vi "io_bin_data_instrument_to_PC.vi"(8 "error in":errorcluster, 10 "Query (none)":string, 11 "VISA resource name":refnum<visa-resource-name>) -> (0 "error out":errorcluster, 1 "Data Size":i32, 2 "String out":string, 3 "VISA resource name out":refnum<visa-resource-name>)   [LabVIEW 2014, in "rszvl_rsidr_core.lvlib"]
uses:
  rszvl_rsidr_core.lvlib
  type_Error_Codes.ctl
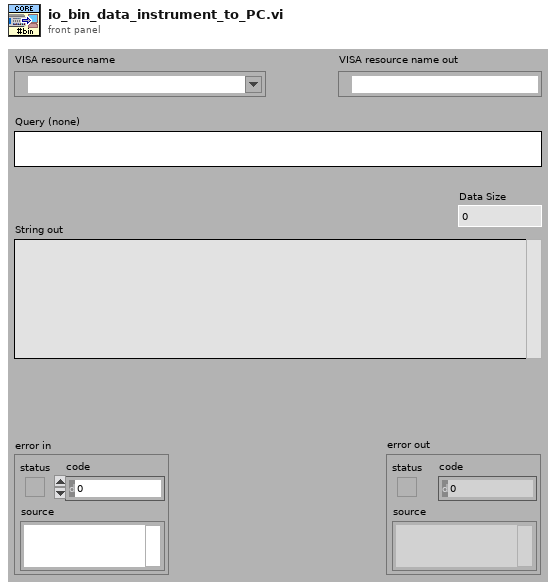
[diagram p1: front panel]
types:
  T1 = typedef "rszvl_rsidr_core.lvlib/type_Error_Codes.ctl" = enum16{"No_error", "VISA_err_ResourceNotFound", "VISA_err_Timeout", "VISA_warn_MoreDataAvailable", "RS_err_MissingCallback", "RS_err_InvalidAttribute", "RS_err_InvalidValue", "RS_err_UnknownResource", "RS_err_AlreadyInitialized", "RS_err_InstrumentStatus", "RS_err_BadRepCapName", "RS_err_TypesMismatch", "RS_err_ValueNotSupported", "RS_err_InvalidRngTable", "RS_err_IDqueryFail", "RS_err_UnexpResponse", "VISA_warn_ConfigNotLoaded", "RS_err_AttributeNotReadable", "RS_err_AttributeNotWritable", "RS_err_InstrumentType", "RS_err_InstrumentOption", "VISA_err_InvalidSize", "RS_err_ReliabilityIndicator", "VISA_warn_UnknownStatus", "VISA_warn_TermCharRead", "VISA_err_IO_error"}
  T2 = typedef "rszvl_rsidr_core.lvlib/type_Session_Data.ctl" = cluster{"Instr type":string, "Instr type for err. msg.":string, "Installed Options":string[], "OPC Timeout":i32, "Query Instrument Status":bool, "Check Range":bool, "Check Options":bool, "Add LF to Write":bool, "Simulate":bool, "Logging":bool, "Logging params":variant, "Interface Type":enum16{"Unknown", "GPIB", "VXI", "GPIB_VXI", "ASRL", "PXI", "TCPIP", "USB", "SOCKET"}, "Fast Sweep":i32, "AdditionalFlags":i32, "WaitBeforeWrite":i32, "WaitBeforeRead":i32, "BinDataChunkSize":i64}
  T3 = enum16{"Unknown", "GPIB", "VXI", "GPIB_VXI", "ASRL", "PXI", "TCPIP", "USB", "SOCKET"}
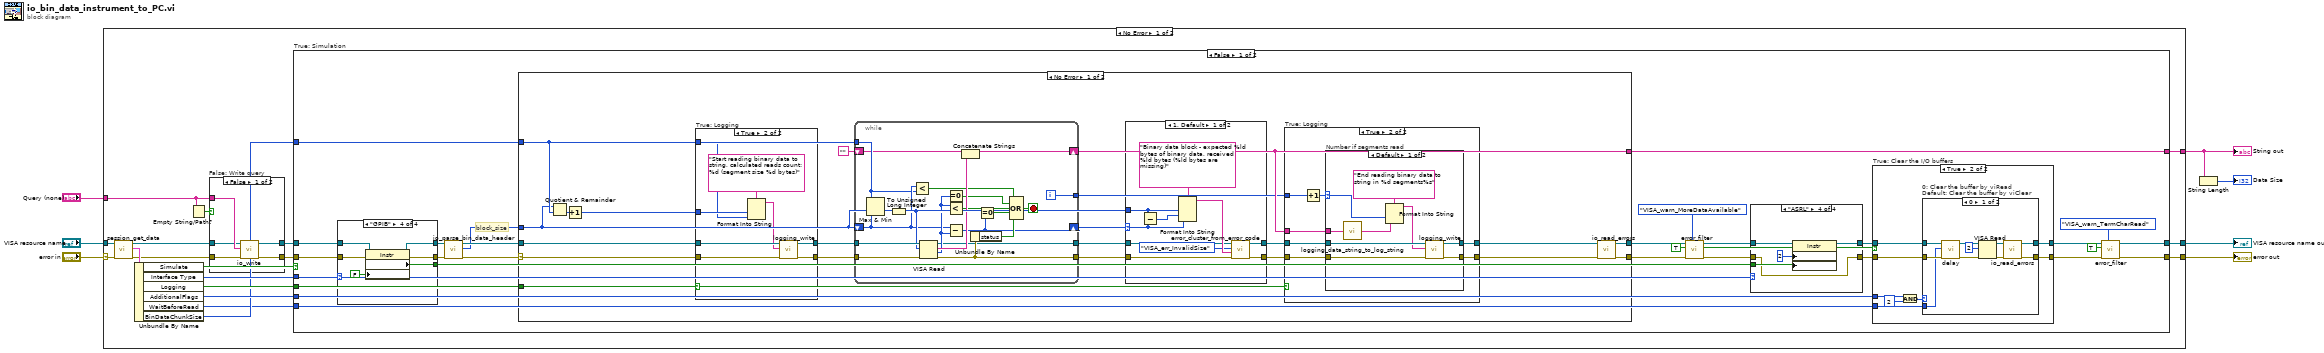
[diagram p0: block diagram]
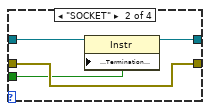
[diagram p4: hidden frame]
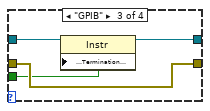
[diagram p5: hidden frame]
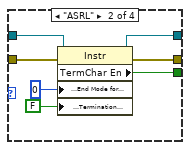
[diagram p7: hidden frame]
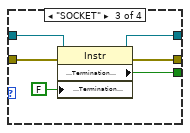
[diagram p8: hidden frame]
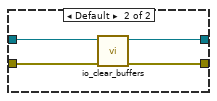
[diagram p10: hidden frame]
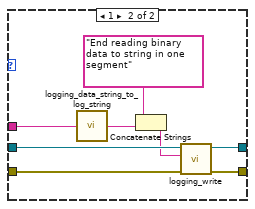
[diagram p12: hidden frame]
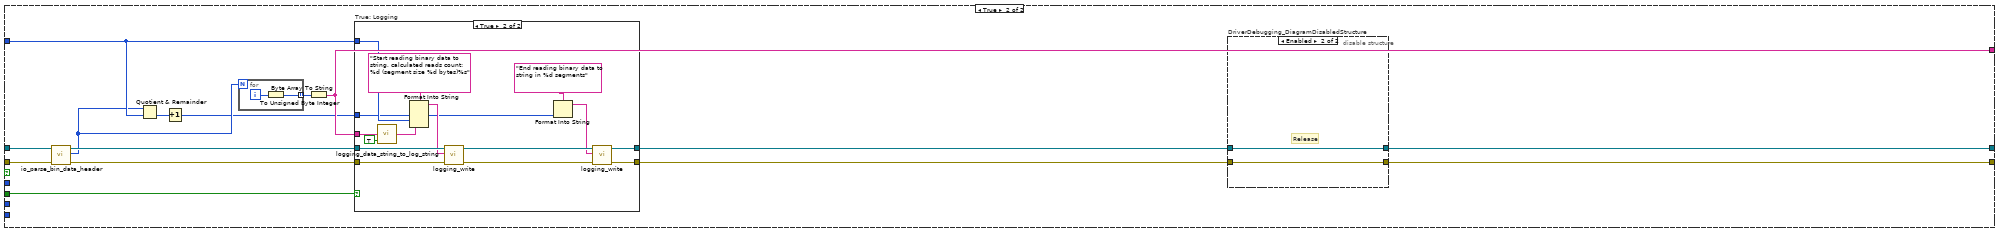
[diagram p16: hidden frame]
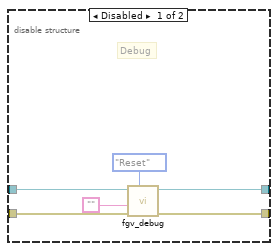
[diagram p18: hidden frame]
diagram:
  n1 = case shown="No Error" "error in" {
    selector: "error in" -> [w23 w256]
    tunnel: [w25 w255] -> w7
    tunnel: [w24 w256] -> w6
    tunnel: "VISA resource name" -> [w22 w255]
    tunnel: [w18 _] -> w2
    tunnel: "Query (none)" -> [w11 _]
    frame No Error {
      n2 = call "session_get_data.vi"("error in"=w23, "VISA resource name"=w22) -> ("error out"=w15:errorcluster, "Session User Data out"=w20:T2, "VISA resource name out"=w14:refnum<visa-resource-name>)  [unwired: 7 in]
      n3 = Unbundle By Name(w20) -> ("Simulate"=w21:bool, "Interface Type"=w19:T3, "Logging"=w17:bool, "AdditionalFlags"=w10:i32, "WaitBeforeRead"=w8:i32, "BinDataChunkSize"=w9:i64)
      n4 = Empty String/Path?(string/path=w11) -> (empty?=w16:bool)
      n5 = case "False: Write query" shown="False" w16 {
        tunnel: w15 -> [w29 w31]
        tunnel: [w27 w31] -> w13
        tunnel: [w26 w32] -> w12
        tunnel: w11 -> [w30 _]
        tunnel: w14 -> [w28 w32]
        frame False {
          n6 = call "io_write.vi"("error in"=w29, "write buffer"=w30, "VISA resource name"=w28) -> ("error out"=w27:errorcluster, "VISA resource name out"=w26:refnum<visa-resource-name>)  [unwired: 7 in]
        }
        frame True {
        }
      }
      n7 = case "True: Simulation" shown="False" w21 {
        tunnel: w13 -> [w48 w225]
        tunnel: w12 -> [w49 w226]
        tunnel: [w38 w214] -> w25
        tunnel: [w37 w215] -> w24
        tunnel: w19 -> [w53 _]
        tunnel: [w52 w219] -> w18
        tunnel: w17 -> [w51 w227]
        tunnel: w9 -> [w50 w222]
        tunnel: w10 -> [w47 _]
        tunnel: w8 -> [w33 _]
        frame False {
          # "block_size"
          n8 = case "4: ASRL" shown="\"GPIB\"" w53 {
            tunnel: w48 -> [w77 w84 w91 w97]
            tunnel: w49 -> [w78 w83 w90 w96]
            tunnel: [w78 w82 w89 w95] -> w57
            tunnel: [w77 w81 w88 w94] -> w58
            tunnel: [_ w79 w86 w92] -> w36
            frame Default {
            }
            frame "ASRL" {
              n9 = property on="Property Node" class="Instr"(reference=w83, error in=w84, "Serial Settings:End Mode for Reads"=u16 0 ("ASRL End In"), "Message Based Settings:Termination Character Enable"=FALSE ("TermChar En")) -> (reference out=w82:refnum<visa-resource-name>, error out=w81:errorcluster, "TermChar En"=w79:bool)
            }
            frame "SOCKET" {
              n10 = property on="Property Node" class="Instr"(reference=w90, error in=w91, "Message Based Settings:Termination Character Enable"=FALSE ("TermChar En")) -> (reference out=w89:refnum<visa-resource-name>, error out=w88:errorcluster, "Message Based Settings:Termination Character Enable"=w86:bool)
            }
            frame "GPIB" {
              n11 = property on="Property Node" class="Instr"(reference=w96, error in=w97, "Message Based Settings:Termination Character Enable"=FALSE ("TermChar En")) -> (reference out=w95:refnum<visa-resource-name>, error out=w94:errorcluster, "Message Based Settings:Termination Character Enable"=w92:bool)
            }
          }
          n12 = call "io_parse_bin_data_header.vi"("error in"=w58, "VISA resource name"=w57) -> ("error out"=w56:errorcluster, "Size of the bin data"=w54:i64, "VISA resource name out"=w55:refnum<visa-resource-name>)  [unwired: 6 in, 1 out]
          n13 = case shown="No Error" w56 {
            selector: w56 -> [w142 w212]
            tunnel: [w137 w212] -> w35
            tunnel: w55 -> [w141 w211]
            tunnel: w54 -> [w131 _]
            tunnel: w50 -> [w134 _]
            tunnel: [w136 w211] -> w34
            tunnel: [w135 _] -> w52
            tunnel: w51 -> [w140 _]
            frame No Error {
              n14 = Quotient & Remainder(x=w131, y=w134) -> (floor(x/y)=w139:i64)  [unwired: 1 out]
              n15 = Increment(x=w139) -> (x+1=w138:i64)
              n16 = case "True: Logging" shown="True" w140 {
                tunnel: w142 -> [w202 w208]
                tunnel: [w202 w210] -> w125
                tunnel: w141 -> [w201 w207]
                tunnel: [w201 w209] -> w126
                tunnel: w134 -> [_ w203]
                tunnel: w138 -> [_ w204]
                frame False {
                }
                frame True {
                  n17 = Format Into String(format string="Start reading binary data to string, calculated reads count: %d (segment size %d bytes)", w204, w203) -> (resulting string=w205:string)  [unwired: 2 in, 1 out]
                  n18 = call "logging_write.vi"("error in"=w208, "String to write"=w205, "VISA resource name"=w207) -> ("error out"=w210:errorcluster, "VISA resource name out"=w209:refnum<visa-resource-name>)  [unwired: 7 in]
                }
              }
              n19 = while {
                tunnel: w125 -> [w186]
                tunnel: w126 -> [w188]
                tunnel: w134 -> [w177]
                shift-right: [w169] -> w127
                shift-left: w131 -> [w178]
                tunnel: [w183] -> w128
                shift-right: [w175] -> w135
                shift-left: "" ("Empty String Constant") -> [w174]
                tunnel: [w173] -> w122
                tunnel: [w172] -> w130
                i -> [w173]
                stop <- w180 stop-if-true
                n20 = Max & Min(x=w177, y=w178) -> (min(x,y)=w187:i64)  [unwired: 1 out]
                n21 = To Unsigned Long Integer(number=w187) -> (unsigned 32bit integer=w184:u32)
                n22 = Less?(x=w178, y=w177) -> (x < y?=w176:bool)
                n23 = VISA Read(VISA resource name=w188, byte count=w184, error in (no error)=w186) -> (VISA resource name out=w172:refnum<visa-resource-name>, read buffer=w185:string, return count=w182:u32, error out=w183:errorcluster)
                n24 = Equal To 0?(x=w182) -> (x = 0?=w179:bool)
                n25 = Less?(x=w182, y=w184) -> (x < y?=w181:bool)
                n26 = Subtract(x=w178, y=w182) -> (x-y=w169:i64)
                n27 = Concatenate Strings(w174, w185) -> (w175:string)
                n28 = Unbundle By Name(w183) -> ("status"=w171:bool)
                n29 = Equal To 0?(x=w169) -> (x = 0?=w170:bool)
                n30 = Compound Arithmetic op=OR(w176, w179, w181, w170, w171) -> (w180:bool)
              }
              n31 = case shown="1, Default" w127 {
                selector: w127 -> [w193 _]
                tunnel: w128 -> [w196 w200]
                tunnel: [w197 w200] -> w123
                tunnel: w131 -> [w195 _]
                tunnel: w130 -> [w190 w199]
                tunnel: [w189 w199] -> w124
                frame 1, Default {
                  n32 = Subtract(x=w195, y=w193) -> (x-y=w194:i64)
                  n33 = Format Into String(format string="Binary data block - expected %ld bytes of binary data, received %ld bytes (%ld bytes are missing)" ("error message (\"\")"), w195, w194, w193) -> (resulting string=w192:string)  [unwired: 2 in, 1 out]
                  n34 = call "error_cluster_from_error_code.vi"("error in"=w196, "error message (\"\")"=w192, "Error Enum in"=type_Error_Codes."VISA_err_InvalidSize", "VISA resource name"=w190) -> ("error out"=w197:errorcluster, "VISA resource name out"=w189:refnum<visa-resource-name>)  [unwired: 6 in]
                }
                frame 0 {
                }
              }
              n35 = case "True: Logging" shown="True" w140 {
                tunnel: w124 -> [w143 w148]
                tunnel: w123 -> [w144 w149]
                tunnel: [w144 w147] -> w132
                tunnel: [w143 w146] -> w133
                tunnel: w122 -> [_ w151]
                tunnel: w135 -> [_ w145]
                frame False {
                }
                frame True {
                  n36 = Increment(x=w151) -> (x+1=w150:i32)
                  n37 = case "Number if segments read" shown="Default" w150 {
                    selector: w150 -> [w154 _]
                    tunnel: w149 -> [w159 w168]
                    tunnel: w148 -> [w158 w167]
                    tunnel: [w157 w166] -> w147
                    tunnel: [w156 w165] -> w146
                    tunnel: w145 -> [w160 w164]
                    frame Default {
                      n38 = call "logging_data_string_to_log_string.vi"("Raw string to log"=w160) -> ("Result log string"=w153:string)  [unwired: 4 in]
                      n39 = Format Into String(format string="End reading binary data to string in %d segments%s", w154, w153) -> (resulting string=w152:string)  [unwired: 2 in, 1 out]
                      n40 = call "logging_write.vi"("error in"=w159, "String to write"=w152, "VISA resource name"=w158) -> ("error out"=w157:errorcluster, "VISA resource name out"=w156:refnum<visa-resource-name>)  [unwired: 7 in]
                    }
                    frame 1 {
                      n41 = call "logging_data_string_to_log_string.vi"("Raw string to log"=w164) -> ("Result log string"=w163:string)  [unwired: 4 in]
                      n42 = Concatenate Strings("End reading binary data to string in one segment" ("format string"), w163) -> (w162:string)
                      n43 = call "logging_write.vi"("error in"=w168, "String to write"=w162, "VISA resource name"=w167) -> ("error out"=w166:errorcluster, "VISA resource name out"=w165:refnum<visa-resource-name>)  [unwired: 7 in]
                    }
                  }
                }
              }
              n44 = call "io_read_errors.vi"("error in"=w132, "VISA resource name"=w133) -> ("error out"=w137:errorcluster, "VISA resource name out"=w136:refnum<visa-resource-name>)  [unwired: 8 in]
            }
            frame Error {
            }
          }
          n45 = call "error_filter.vi"("Error Enum in"=type_Error_Codes."VISA_warn_MoreDataAvailable" ("Code to detect"), "error in"=w35, "Clear detected code (F)"=TRUE ("Clear detected error (F)"), "VISA resource name"=w34) -> ("error out"=w45:errorcluster, "Code Detected"=w61:bool, "VISA resource name out"=w46:refnum<visa-resource-name>)  [unwired: 5 in]
          n46 = case "4: ASRL" shown="\"ASRL\"" w53 {
            tunnel: w46 -> [w63 w67 w71 w74]
            tunnel: [w63 w66 w70 w75] -> w44
            tunnel: w45 -> [w62 w65 w69 w72]
            tunnel: [w62 w65 w69 w72] -> w43
            tunnel: w36 -> [_ w64 w68 w73]
            frame Default {
            }
            frame "SOCKET" {
              n47 = property on="Property Node" class="Instr"(reference=w67, "Message Based Settings:Termination Character Enable"=w64) -> (reference out=w66:refnum<visa-resource-name>)  [unwired: 1 in, 1 out]
            }
            frame "GPIB" {
              n48 = property on="Property Node" class="Instr"(reference=w71, "Message Based Settings:Termination Character Enable"=w68) -> (reference out=w70:refnum<visa-resource-name>)  [unwired: 1 in, 1 out]
            }
            frame "ASRL" {
              n49 = property on="Property Node" class="Instr"(reference=w74, "Serial Settings:End Mode for Reads"=u16 2 ("ASRL End In"), "Message Based Settings:Termination Character Enable"=w73) -> (reference out=w75:refnum<visa-resource-name>)  [unwired: 1 in, 1 out]
            }
          }
          n50 = case "True: Clear the I/O buffers" shown="True" w61 {
            tunnel: [w98 w105] -> w39
            tunnel: w44 -> [w99 w106]
            tunnel: w43 -> [w98 w107]
            tunnel: [w99 w104] -> w40
            tunnel: w47 -> [_ w103]
            tunnel: w33 -> [_ w100]
            frame False {
            }
            frame True {
              n51 = And(x=w103, y=2 ("x")) -> (x .and. y?=w102:i32)
              n52 = case "0: Clear the buffer by viRead\nDefault: Clear the buffer by viClear" shown="0" w102 {
                tunnel: w107 -> [w112 w121]
                tunnel: w106 -> [w111 w120]
                tunnel: [w114 w119] -> w105
                tunnel: [w113 w118] -> w104
                tunnel: w100 -> [w108 _]
                frame 0 {
                  n53 = call "delay.vi"("error in"=w112, "Milliseconds to wait"=w108, "VISA resource name"=w111) -> ("error out"=w110:errorcluster, "VISA resource name out"=w109:refnum<visa-resource-name>)  [unwired: 7 in]
                  n54 = VISA Read ("Read the junk")(VISA resource name=w109, byte count=u32 2, error in (no error)=w110) -> (VISA resource name out=w115:refnum<visa-resource-name>, error out=w116:errorcluster)  [unwired: 2 out]
                  n55 = call "io_read_errors.vi"("error in"=w116, "VISA resource name"=w115) -> ("error out"=w114:errorcluster, "VISA resource name out"=w113:refnum<visa-resource-name>)  [unwired: 8 in]
                }
                frame Default {
                  n56 = call "io_clear_buffers.vi"("error in"=w121, "VISA resource name"=w120) -> ("error out"=w119:errorcluster, "VISA resource name out"=w118:refnum<visa-resource-name>)  [unwired: 8 in]
                }
              }
            }
          }
          n57 = call "error_filter.vi"("Error Enum in"=type_Error_Codes."VISA_warn_TermCharRead", "error in"=w39, "Clear detected code (F)"=TRUE, "VISA resource name"=w40) -> ("error out"=w37:errorcluster, "VISA resource name out"=w38:refnum<visa-resource-name>)  [unwired: 5 in, 1 out]
        }
        frame True {
          n58 = call "io_parse_bin_data_header.vi"("error in"=w225, "VISA resource name"=w226) -> ("error out"=w223:errorcluster, "Size of the bin data"=w220:i64, "VISA resource name out"=w224:refnum<visa-resource-name>)  [unwired: 6 in, 1 out]
          n59 = Quotient & Remainder(x=w220, y=w222) -> (floor(x/y)=w221:i64)  [unwired: 1 out]
          n60 = Increment(x=w221) -> (x+1=w218:i64)
          n61 = for {
            N: w220 -> [_]
            tunnel: [w228] -> w213 mode=indexing
            i -> [w229]
            n62 = To Unsigned Byte Integer(number=w229) -> (unsigned 8bit integer=w228:u8)
          }
          n63 = Byte Array To String(unsigned byte array=w213) -> (string=w219:string)
          n64 = case "True: Logging" shown="True" w227 {
            tunnel: w223 -> [w231 w246]
            tunnel: [w231 w238] -> w216
            tunnel: w224 -> [w230 w245]
            tunnel: [w230 w239] -> w217
            tunnel: w222 -> [_ w242]
            tunnel: w218 -> [_ w236]
            tunnel: w219 -> [_ w233]
            frame False {
            }
            frame True {
              n65 = call "logging_data_string_to_log_string.vi"("Force binary format (F)"=TRUE, "Raw string to log"=w233) -> ("Result log string"=w234:string)  [unwired: 3 in]
              n66 = Format Into String(format string="Start reading binary data to string, calculated reads count: %d (segment size %d bytes)%s", w236, w242, w234) -> (resulting string=w243:string)  [unwired: 2 in, 1 out]
              n67 = call "logging_write.vi"("error in"=w246, "String to write"=w243, "VISA resource name"=w245) -> ("error out"=w240:errorcluster, "VISA resource name out"=w241:refnum<visa-resource-name>)  [unwired: 7 in]
              n68 = Format Into String(format string="End reading binary data to string in %d segments", w236) -> (resulting string=w235:string)  [unwired: 2 in, 1 out]
              n69 = call "logging_write.vi"("error in"=w240, "String to write"=w235, "VISA resource name"=w241) -> ("error out"=w238:errorcluster, "VISA resource name out"=w239:refnum<visa-resource-name>)  [unwired: 7 in]
            }
          }
          n70 = disable-structure "DriverDebugging_DiagramDisabledStructure" shown="Enabled" {
            disable-tunnel: w216 -> [w251 w253]
            disable-tunnel: [w249 w253] -> w215
            disable-tunnel: w217 -> [w250 w254]
            disable-tunnel: [w248 w254] -> w214
            frame Disabled {
              # "Debug"
              n71 = call "fgv_debug.vi"("Operation"=enum16{"Reset", "ReadCommand", "SetCommand"}."Reset", "error in"=w251, "Command in"="" ("Empty String Constant"), "VISA resource name"=w250) -> ("error out"=w249:errorcluster, "VISA resource name out"=w248:refnum<visa-resource-name>)  [unwired: 6 in]
            }
            frame Enabled {
              # "Release"
            }
          }
        }
      }
    }
    frame Error {
    }
  }
  "error out" <- w6
  "VISA resource name out" <- w7
  "String out" <- w2
  n72 = String Length(string=w2) -> (length=→"Data Size":i32)
